vi "MDF4 Add Channel Group.vi"(6 "Record ID":u64, 7 "path in":path, 8 "Error In":errorcluster, 9 "chan_count":u32, 10 "Data Group Reference in":i64, 11 "MDF4 File Reference in":i64) -> (0 "Error Out":errorcluster, 1 "Channel Group Reference out":i64, 2 "Data Group Reference out":i64, 3 "MDF4 File Reference out":i64)   [LabVIEW 2019, in "MD4Logger Engine.lvlib"]
uses:
  MD4Logger Engine.lvlib
  <vilib>/Utility/error.llb/Error Cluster From Error Code.vi
  <vilib>/ErrorRing/Error Ring.xnode
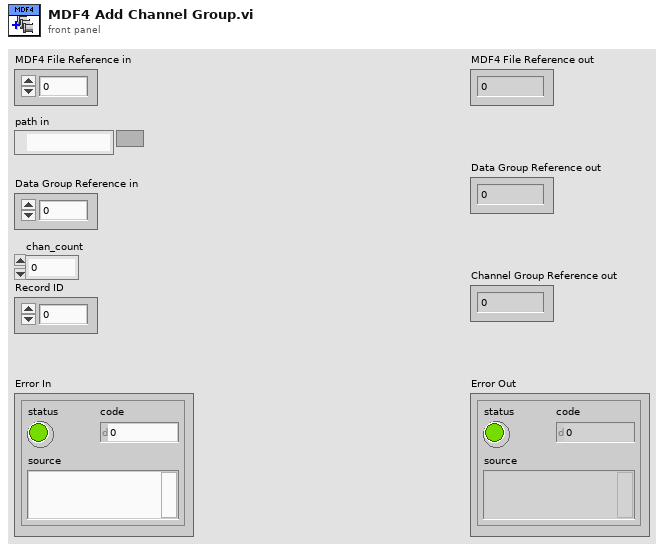
[diagram p1: front panel]
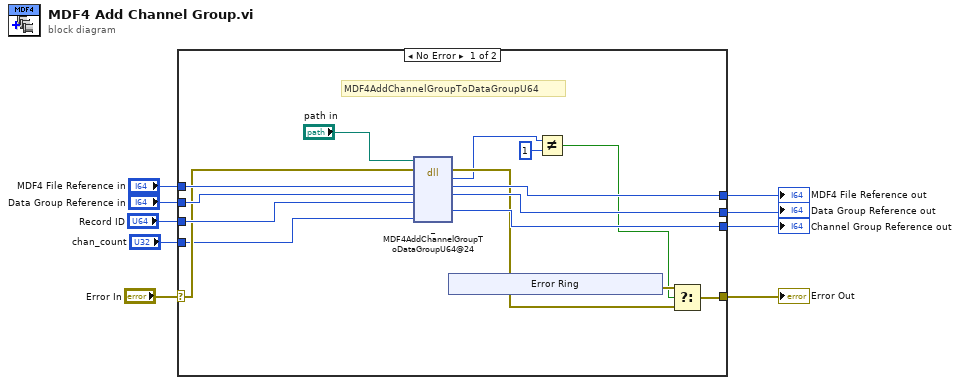
[diagram p0: block diagram]
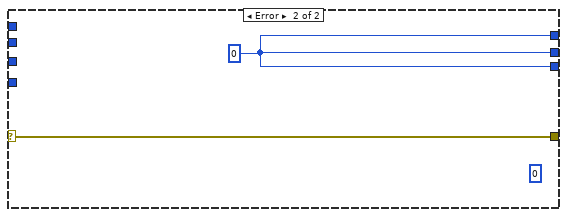
[diagram p2: hidden frame]
diagram:
  n1 = case shown="No Error" "Error In" {
    selector: "Error In" -> [w15 w31]
    tunnel: "MDF4 File Reference in" -> [w24 _]
    tunnel: [w16 w31] -> w7
    tunnel: [w23 w30] -> w6
    tunnel: [w22 w30] -> w5
    tunnel: "Data Group Reference in" -> [w21 _]
    tunnel: [w20 w30] -> w3
    tunnel: "Record ID" -> [w17 _]
    tunnel: "chan_count" -> [w10 _]
    frame No Error {
      # "MDF4AddChannelGroupToDataGroupU64"
      n2 = dll-call lib="C:/Users/Hovhannes/Desktop/MD4Logger/Source/Engine/DLL/WriterExample.dll" fn="_MDF4AddChannelGroupToDataGroupU64@24"(path in="path in", error in=w15, "m4"=w24, "dg"=w21, "rec_id"=w17, "chan_count"=w10) -> (error out=w18:errorcluster, "return type"=w13:i32, "m4"=w22:i64, "dg"=w23:i64, "cg"=w20:i64)  [unwired: 4 in, 1 out]
      n3 = xnode "Error Ring"() -> ("error out"=w19:errorcluster)
      n4 = Not Equal?(x=w13, y=1) -> (x != y?=w12:bool)
      n5 = Select(t=w19, s=w12, f=w18) -> (s? t:f=w16:errorcluster)
    }
    frame Error {
      (unwired) u32 0 ("byte_count")
      w30 = i64 0 ("m4")
    }
  }
  "Data Group Reference out" <- w6
  "Error Out" <- w7
  "MDF4 File Reference out" <- w5
  "Channel Group Reference out" <- w3
